vi "Dialog - File Already Exists.vi"(4 "Error In":errorcluster, 6 "Message In":string) -> (0 "Error Out":errorcluster, 1 "Do same for all":bool, 3 "Selected Button":T1=enum."Copy")   [LabVIEW 2018]
uses:
  Dialog Buttons.ctl
panel:
  in  "Do same for all":bool caption="Do same for all init val"
  in  "Button Cluster":T1
  # "+"
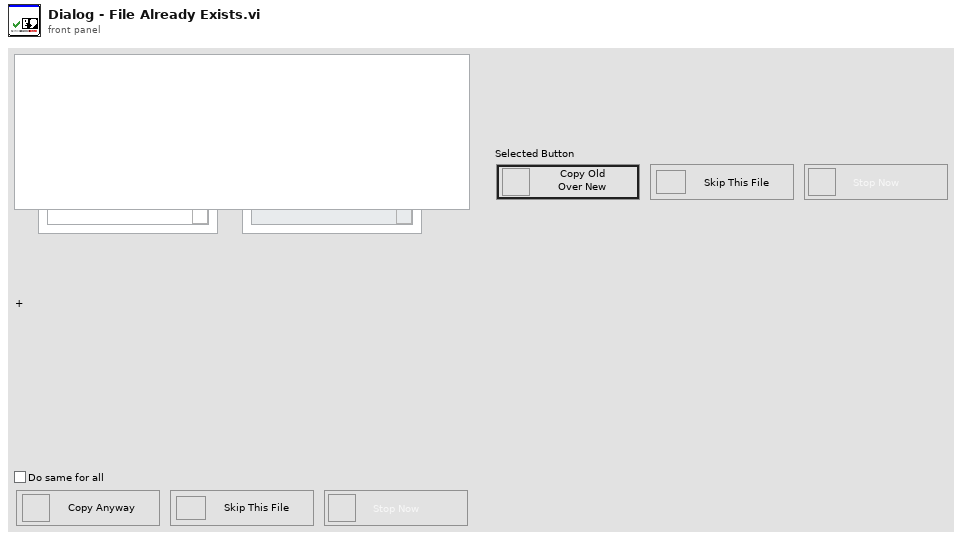
[diagram p1: front panel]
types:
  T1 = typedef "Dialog Buttons.ctl" = enum32{"No Selection", "Copy", "Skip Ahead", "Stop"}
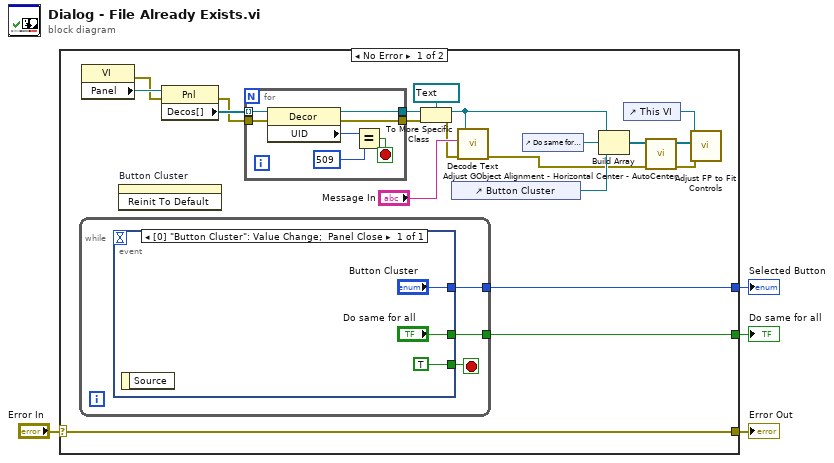
[diagram p0: block diagram]
diagram:
  n1 = case shown="No Error" "Error In" {
    selector: "Error In" -> [w24 w38]
    tunnel: [w24 w38] -> w3
    tunnel: [w22 _] -> w2
    tunnel: [w23 _] -> w1
    frame No Error {
      n2 = while {
        tunnel: [w33] -> w22
        tunnel: [w32] -> w23
        stop <- w34 stop-if-true
        n3 = event shown="[0] \"Button Cluster\": Value Change;  Panel Close" {
          selector: _ -> [_]
          dyn-events: _ -> [_]
          timeout: _ -> [_]
          tunnel: [TRUE] -> w34
          tunnel: ["Button Cluster"] -> w33
          tunnel: ["Do same for all"] -> w32
          event Value Change; Panel Close {
            n4 = event-data() -> ()  [unwired: 1 in, 1 out]
          }
        }
      }
      n5 = property class="VI"() -> (error out=w17:errorcluster, "Panel"=w20:refnum<vi>)  [unwired: 2 in, 1 out]
      n6 = invoke on="Button Cluster" class="RadioBtnsControl (strict)" method="Reinit To Default"() -> ()  [unwired: 3 in, 3 out]
      n7 = property on="Property Node" class="Pnl"(reference=w20, error in=w17) -> (error out=w18:errorcluster, "Decos[]"=w19:refnum<vi>[])  [unwired: 1 out]
      n8 = for {
        tunnel: w19 -> [w31] mode=indexing
        tunnel: [w28] -> w16
        tunnel: [w26] -> w14
        tunnel: w18 -> [w25]
        stop <- w27 stop-if-true
        n9 = property on="Property Node" class="Decor"(reference=w31, error in=w25) -> (reference out=w28:refnum<vi>, error out=w26:errorcluster, "UID"=w30:i32)
        n10 = Equal?(x=w30, y=509 ("UID")) -> (x = y?=w27:bool)
      }
      n11 = To More Specific Class(target class=refnum<vi> refnum ("reference"), reference=w16, error in=w14) -> (specific class reference=w12:refnum<vi>, error out=w13:errorcluster)
      n12 = control-ref of="Button Cluster"() -> (w10:refnum<vi>)
      n13 = call "Decode Text.vi"("error in"=w13, "Encoded String"="Message In", "Text Ref"=w12) -> ("error out"=w6:errorcluster)  [unwired: 3 in, 1 out]
      n14 = control-ref of="Do same for all"() -> (w11:refnum<vi>)
      n15 = Build Array(w12, w11, w10) -> (w9:refnum<vi>[])
      n16 = control-ref of="This VI"() -> (w7:refnum<vi>)
      n17 = call "Adjust GObject Alignment - Horizontal Center - AutoCenter.vi"("error in"=w6, "GObj Refs"=w9) -> ("error out"=w5:errorcluster, "dup GObj Refs"=w8:refnum<vi>[])  [unwired: 4 in]
      n18 = call "Adjust FP to Fit Controls.vi"("Error In"=w5, "Controls & Decorations"=w8, "VI ref"=w7) -> ()  [unwired: 5 in, 2 out]
    }
    frame Error {
    }
  }
  "Error Out" <- w3
  "Selected Button" <- w2
  "Do same for all" <- w1
